vi "Cumulative Per Shift.vi"(10 "Current Hour Index":i32, 11 "Shift Hour Data":u32[][](array[numeric])) -> (2 "Target Cummulative Per Hour":u32, 3 "Target Cummulative Per Shift":u32)   [LabVIEW 2018]
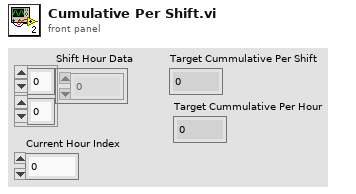
[diagram p1: front panel]
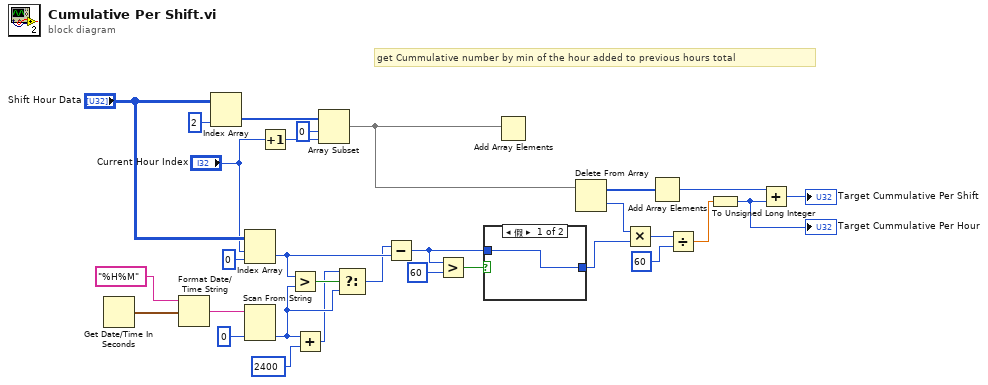
[diagram p0: block diagram]
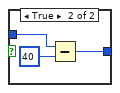
[diagram p2: hidden frame]
diagram:
  # "get Cummulative number by min of the hour added to previous hours total"
  n1 = Get Date/Time In Seconds() -> (seconds since 1Jan1904=w19:timestamp)
  n2 = Format Date/Time String(time format string (%c)="%H%M", seconds (now)=w19) -> (date/time string=w21:string)  [unwired: 1 in]
  n3 = Index Array(array="Shift Hour Data", index (col)=2 ("disabled index (col)")) -> (element=w29:u32[])  [unwired: 1 in]
  n4 = Index Array(array="Shift Hour Data", index (row)="Current Hour Index", index (col)=0 ("disabled index (col)")) -> (element=w8:u32)
  n5 = Scan From String(input string=w21, default 1=u32 0) -> (output 1=w5:u32)  [unwired: 3 in, 3 out]
  n6 = Increment(x="Current Hour Index") -> (x+1=w30:i32)
  n7 = Greater?(x=w8, y=w5) -> (0:w7:bool)
  n8 = Add(x=w5, y=u32 2400) -> (x+y=w3:u32)
  n9 = Array Subset(array=w29, index=0, length=w30) -> (w1:u32[])
  n10 = Select(t=w3, s=w7, f=w5) -> (s? t:f=w6:u32)
  n11 = Subtract(x=w6, y=w8) -> (x-y=w11:u32)
  n12 = Greater?(x=w11, y=u32 60) -> (0:w12:bool)
  n13 = case shown="假" w12 {
    tunnel: w11 -> [w31 w34]
    tunnel: [w31 w32] -> w9
    frame False {
    }
    frame True {
      n14 = Subtract(x=w34, y=u32 40) -> (x-y=w32:u32)
    }
  }
  n15 = Add Array Elements(numeric array=w1) -> ()  [unwired: 1 out]
  n16 = Delete From Array(array=w1) -> (deleted portion=w18:u32, array with subset deleted=w26:u32[])  [unwired: 2 in]
  n17 = Multiply(x=w18, y=w9) -> (x*y=w17:u32)
  n18 = Add Array Elements(numeric array=w26) -> (sum=w15:u32)
  n19 = Divide(x=w17, y=u32 60) -> (x/y=w14:dbl)
  n20 = To Unsigned Long Integer(number=w14) -> (unsigned 32bit integer=w13:u32)
  "Target Cummulative Per Hour" <- w13
  n21 = Add(x=w15, y=w13) -> (x+y=→"Target Cummulative Per Shift":u32)
